vi "Read Error.vi"(11 "Error in":refnum<class "Error.lvclass">) -> (2 "Error":errorcluster, 3 "Error out":refnum<class "Error.lvclass">)   [LabVIEW 2021, in "jettl.lvlib" / "Error.lvclass"]
uses:
  Error.lvclass
  Error.lvclass/Error.ctl
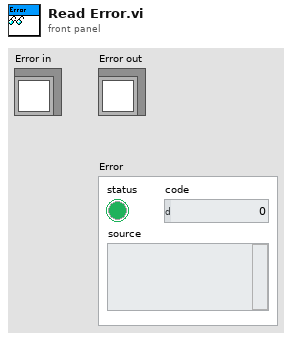
[diagram p1: front panel]
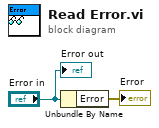
[diagram p0: block diagram]
diagram:
  n1 = Unbundle By Name("Error in") -> ("Error"=→"Error":errorcluster)
  "Error out" <- "Error in"
